vi "ZLIB Extract File__ogtk.vi"(4 "password (none)":string, 5 "overwrite (F)":bool, 6 "error in (no error)":errorcluster, 7 "internal name (same as target)":string, 8 "target path":path, 9 "unzip Refnum":T1) -> (0 "error out":errorcluster, 3 "unzip Refnum out":T1)   [LabVIEW 2012]
doc: "Extracts a file in an unzip session to a target path."
uses:
  <userlib>/_OpenG.lib/lvzip/lvzip.llb/ZLIB Unzip Handle__ogtk.ctl
panel:
  # "Please visit http://www.OpenG.org to learn about the\nOpen Source LabVIEW software movement.\n\nNOTICE -- YOU MUST LEAVE THIS NOTICE IN PLACE.  PER THE TERMS OF THE LICENSE BELOW, YOU MAY SUBLICENSE THIS SOFTWARE \nIN ANY WAY THAT DOES NOT CONFLICT WITH THIS LICENSE.\n\n### BSD License (http://www.opensource.org/licenses/bsd-license.php) Begin ###\n \nCopyright (C) 2002 Rolf Kalbermatter rolf.kalbermatter@citeng.com\nCopyright (C) 2002 Jim Kring jim@jimkring.com\n\nAll rights reserved.\n\nRedistribution and use in source and binary forms, with or without modification, are permitted provided that the following conditions are met:\n\n    * Redistributions of source code must retain the above copyright notice, this list of conditions and the following disclaimer.\n    * Redistributions in binary form must reproduce the above copyright notice, this list of conditions and the following disclaimer in the \n       documentation and/or other materials provided with the distribution.\n    * Neither the name of SciWare, James Kring, Inc., nor the names of its contributors may be used to endorse or promote products derived \n       from this software without specific prior written permission.\n\nTHIS SOFTWARE IS PROVIDED BY THE COPYRIGHT HOLDERS AND CONTRIBUTORS \"AS IS\" AND ANY EXPRESS OR IMPLIED WARRANTIES, \nINCLUDING, BUT NOT LIMITED TO, THE IMPLIED WARRANTIES OF MERCHANTABILITY AND FITNESS FOR A PARTICULAR PURPOSE ARE \nDISCLAIMED. IN NO EVENT SHALL THE COPYRIGHT OWNER OR CONTRIBUTORS BE LIABLE FOR ANY DIRECT, INDIRECT, INCIDENTAL,\n SPECIAL, EXEMPLARY, OR CONSEQUENTIAL DAMAGES (INCLUDING, BUT NOT LIMITED TO, PROCUREMENT OF SUBSTITUTE GOODS OR \nSERVICES; LOSS OF USE, DATA, OR PROFITS; OR BUSINESS INTERRUPTION) HOWEVER CAUSED AND ON ANY THEORY OF LIABILITY, \nWHETHER IN CONTRACT, STRICT LIABILITY, OR TORT (INCLUDING NEGLIGENCE OR OTHERWISE) ARISING IN ANY WAY OUT OF THE USE \nOF THIS SOFTWARE, EVEN IF ADVISED OF THE POSSIBILITY OF SUCH DAMAGE.\n\n### BSD License End ###"
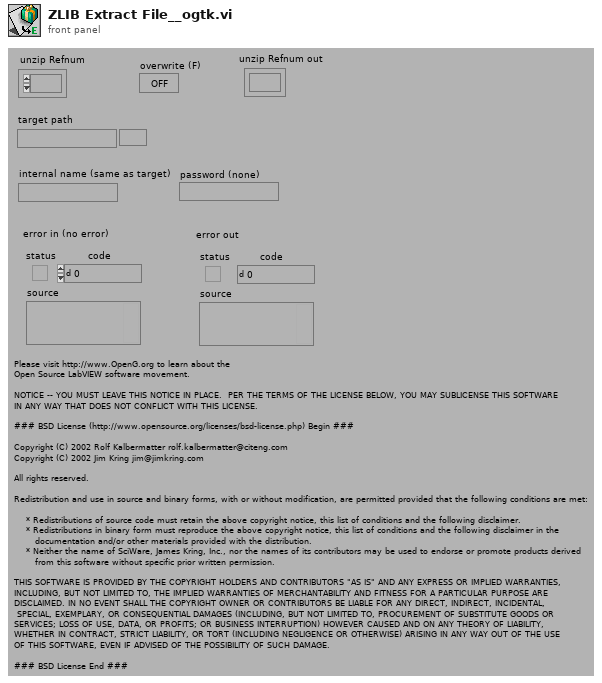
[diagram p1: front panel]
types:
  T1 = typedef "ZLIB Unzip Handle__ogtk.ctl" = refnum<k1>
  T2 = typedef "ZLIB File Info__ogtk.ctl" = cluster{"version":u32, "version needed":u32, "encrypted":bool, "flag":u32, "compression":i32, "dos date":u32, "crc":u32, "compressed size":u32, "uncompressed size":u32, "extra info":string, "file comment":string, "disk num start":u32, "internal fa":u32, "external fa":u32, "file timestamp":u32}
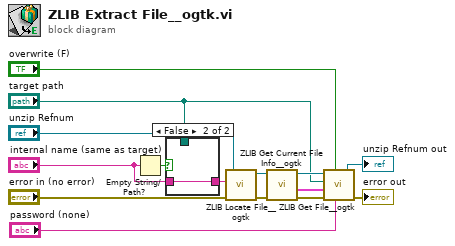
[diagram p0: block diagram]
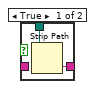
[diagram p2: hidden frame]
diagram:
  n1 = Empty String/Path?(string/path="internal name (same as target)") -> (empty?=w3:bool)
  n2 = case shown="False" w3 {
    tunnel: "target path" -> [w17 _]
    tunnel: [w16 w18] -> w6
    tunnel: "internal name (same as target)" -> [_ w18]
    frame True {
      n3 = Strip Path(path=w17) -> (name=w16:string)  [unwired: 1 out]
    }
    frame False {
    }
  }
  n4 = call <userlib>:"ZLIB Locate File__ogtk.vi"("error in (no error)"="error in (no error)", "name (empty: -)"=w6, "unzip Refnum"="unzip Refnum") -> ("error out"=w10:errorcluster, "unzip Refnum out"=w15:T1)  [unwired: 3 in]
  n5 = call <userlib>:"ZLIB Get Current File Info__ogtk.vi"("error in (no error)"=w10, "unzip Refnum"=w15) -> ("error out"=w14:errorcluster, "file info"=w1:T2, "unzip Refnum out"=w13:T1)  [unwired: 6 in, 1 out]
  n6 = call <userlib>:"ZLIB Get File__ogtk.vi"("password (none)"="password (none)", "overwrite (F)"="overwrite (F)", "error in (no error)"=w14, "file info"=w1, "target path"="target path", "unzip Refnum"=w13) -> ("error out"=→"error out":errorcluster, "unzip Refnum out"=→"unzip Refnum out":T1)  [unwired: 2 in]
